vi "Create Table.vi"(8 "error in (no error)":errorcluster, 10 "Primary Key?":bool=TRUE, 11 "SQLObject in":refnum<class "SQLObject.lvclass">) -> (0 "error out":errorcluster, 3 "SQLObject out":refnum<class "SQLObject.lvclass">)   [LabVIEW 2021, in "SQLObject.lvclass"]
uses:
  SQLObject.lvclass
  SQLObject.lvclass/SQLObject.ctl
  <vilib>/drjdpowell/SQLite Library/SQL Connection/Execute SQL (No results).vi
  <vilib>/drjdpowell/SQLite Library/SQLite.lvlib
  <vilib>/drjdpowell/SQLite Library/SQL Connection/Connection.lvclass
panel:
  out "SQL QUERY":string
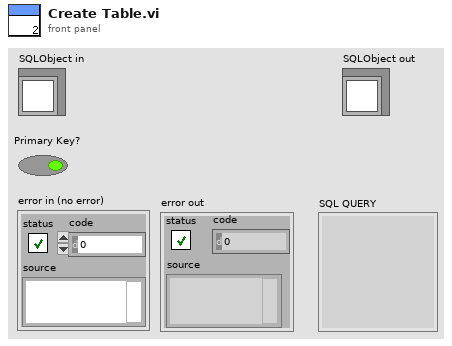
[diagram p1: front panel]
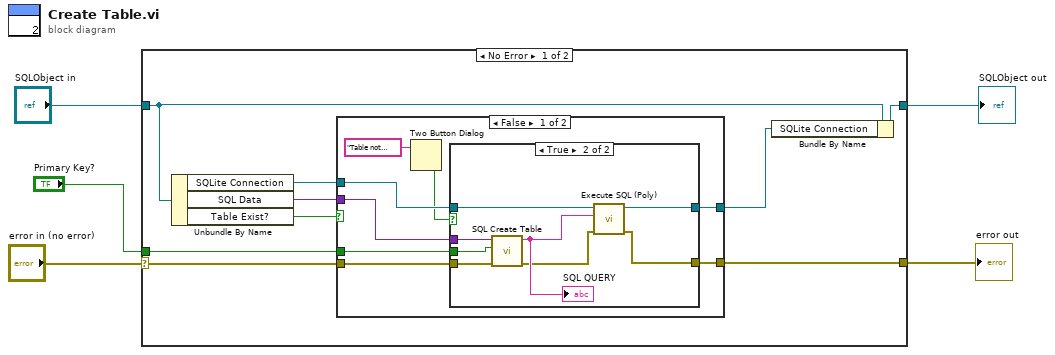
[diagram p0: block diagram]
diagram:
  n1 = case shown="No Error" "error in (no error)" {
    selector: "error in (no error)" -> [w14 w36]
    tunnel: [w13 w36] -> w4
    tunnel: [w6 w35] -> w2
    tunnel: "SQLObject in" -> [w8 w35]
    tunnel: "Primary Key?" -> [w9 _]
    frame No Error {
      n2 = Unbundle By Name(w8) -> ("SQLite Connection"=w11:refnum<class "Connection.lvclass">, "SQL Data"=w12:variant, "Table Exist?"=w10:bool)
      n3 = case shown="False" w10 {
        tunnel: w14 -> [w22 w34]
        tunnel: [w21 w34] -> w13
        tunnel: w12 -> [w19 _]
        tunnel: w11 -> [w20 w33]
        tunnel: w9 -> [w16 _]
        tunnel: [w15 w33] -> w7
        frame False {
          n4 = Two Button Dialog(message="Table not found in database will be recreated") -> (T button?=w17:bool)  [unwired: 2 in]
          n5 = case shown="True" w17 {
            tunnel: w22 -> [w24 w31]
            tunnel: [w24 w29] -> w21
            tunnel: w20 -> [w23 w28]
            tunnel: w19 -> [_ w27]
            tunnel: w16 -> [_ w26]
            tunnel: [w23 w25] -> w15
            frame False {
            }
            frame True {
              n6 = call "SQL Create Table.vi"("error in"=w31, "Primary Key?"=w26, "variant"=w27) -> ("error out"=w30:errorcluster, "SQL QUERY"=w32:string)  [unwired: 6 in, 1 out]
              "SQL QUERY" <- w32
              n7 = call-poly <vilib>:"Execute SQL (Poly).vi"("error in (no error)"=w30, "SQL"=w32, "SQLite Connection in"=w28) -> ("error out"=w29:errorcluster, "SQLite Connection"=w25:refnum<class "Connection.lvclass">)  [unwired: 7 in]
            }
          }
        }
        frame True {
        }
      }
      n8 = Bundle By Name(cluster=w8, "SQLite Connection"=w7) -> (w6:refnum<class "SQLObject.lvclass">)
    }
    frame Error {
    }
  }
  "error out" <- w4
  "SQLObject out" <- w2
